vi "Return to Normal.vi"(8 "error in (no error)":errorcluster, 11 "Data Cluster in":T1 {"VestaTemperature"."Water Heater Temp (°F)" min=32 max=203}) -> (0 "error out":errorcluster, 1 "Send_Vesta_Message":u8, 3 "Data Cluster Output":T1 {"VestaTemperature"."Water Heater Temp (°F)" min=32 max=203})   [LabVIEW 2023]
uses:
  Drivers/Resideo Gas Valve/Type Definitions/Temperature Control.ctl
  Message Queue/Message Queue.lvlib
  Message Queue/Enqueue Message (Single).vi
  Drivers/Resideo Gas Valve/Type Definitions/Vesta Info.ctl
  controls/Burner Duty Cycle.ctl
  controls/Timer Application Cluster.ctl
  controls/UI Data.ctl
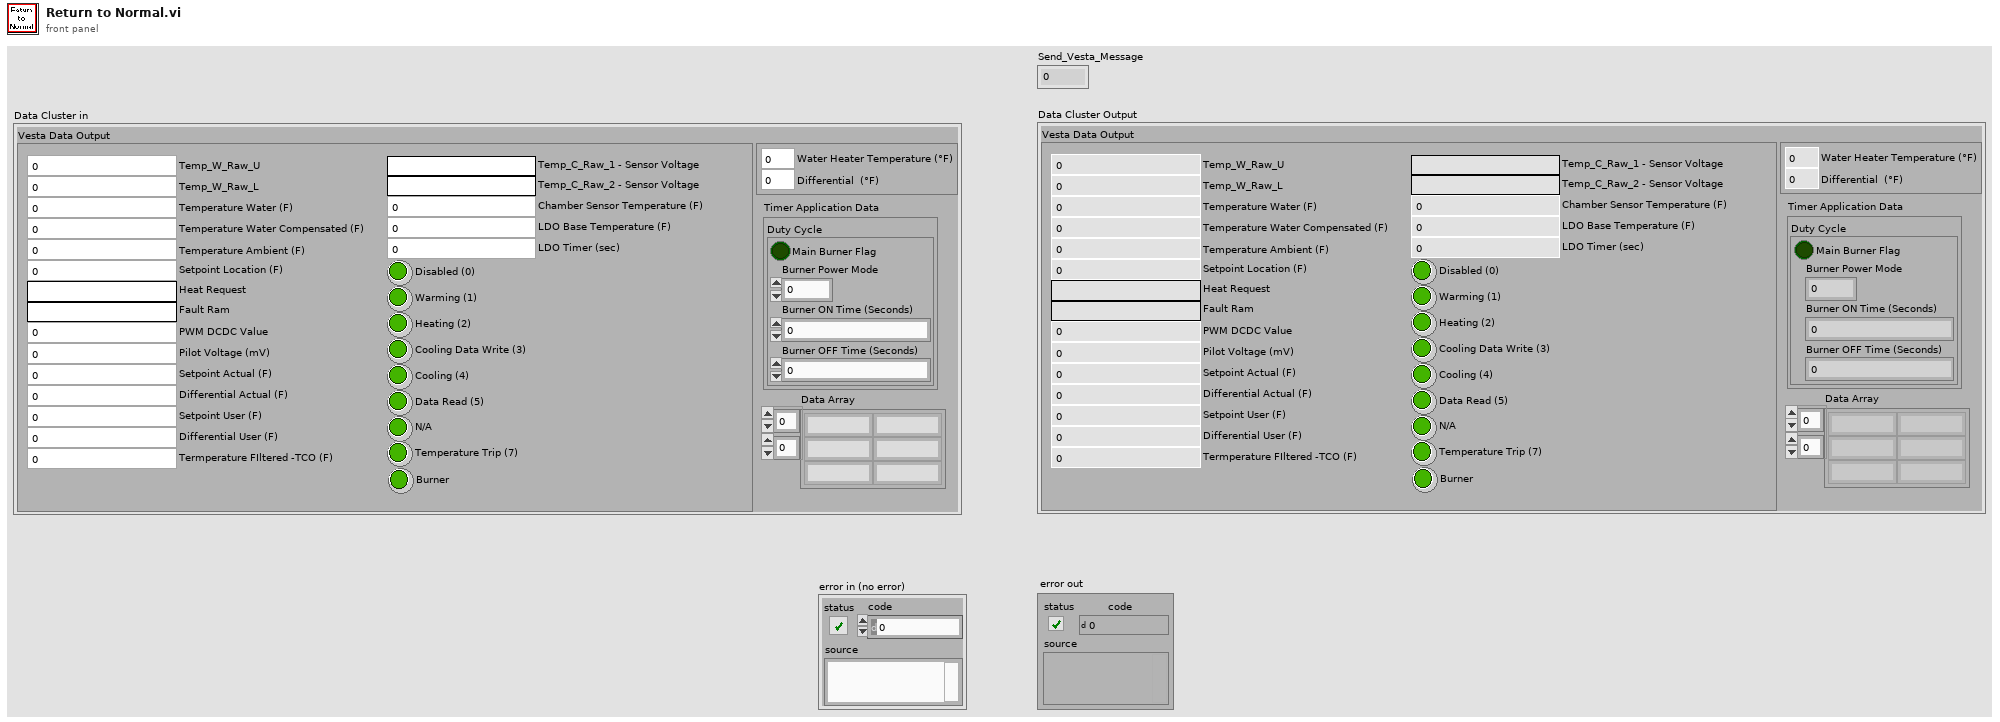
[diagram p1: front panel]
types:
  T1 = typedef "UI Data.ctl" = cluster{"Vesta Data Output":T2, "VestaTemperature":T3, "Timer Application Data":T4, "Data Array":string[][]}
  T2 = typedef "Vesta Info.ctl" = cluster{"Temp_W_Raw_U":u16, "Temp_W_Raw_L":u16, "Temperature Water (F)":dbl, "Temperature Water Compensated (F)":dbl, "Temperature Ambient (F)":dbl, "Setpoint Location (F)":dbl, "Heat Request":string, "Fault Ram":string, "PWM DCDC Value":u16, "Pilot Voltage (mV)":dbl, "Setpoint Actual (F)":dbl, "Differential Actual (F)":dbl, "Setpoint User (F)":dbl, "Differential User (F)":dbl, "Termperature FIltered -TCO (F)":dbl, "Temp_C_Raw_1 - Sensor Voltage":string, "Temp_C_Raw_2 - Sensor Voltage":string, "Chamber Sensor Temperature (F)":dbl, "LDO Base Temperature (F)":dbl, "LDO Timer (sec)":i16, "Disabled (0)":bool, "Warming (1)":bool, "Heating (2)":bool, "Cooling Data Write (3)":bool, "Cooling (4)":bool, "Data Read (5)":bool, "N/A":bool, "Temperature Trip (7)":bool, "Burner":bool}
  T3 = typedef "Temperature Control.ctl" = cluster{"Water Heater Temp (°F)":u16, "Differential  (°F)":dbl}
  T4 = typedef "Timer Application Cluster.ctl" = cluster{"Duty Cycle":T5}
  T5 = typedef "Burner Duty Cycle.ctl" = cluster{"Burner ON Time (Seconds)":dbl, "Burner OFF Time (Seconds)":dbl, "Main Burner Flag":bool, "Burner Power Mode":u8}
  T6 = typedef "UI Data.ctl" = cluster{"Vesta Data Output":T2, "VestaTemperature":T3, "Timer Application Data":T7}
  T7 = typedef "Timer Application Cluster.ctl" = cluster{"Time Data":T8, "Duty Cycle":T5}
  T8 = typedef "Timers.ctl" = cluster{"Main Timer":dbl, "Burner Status":bool}
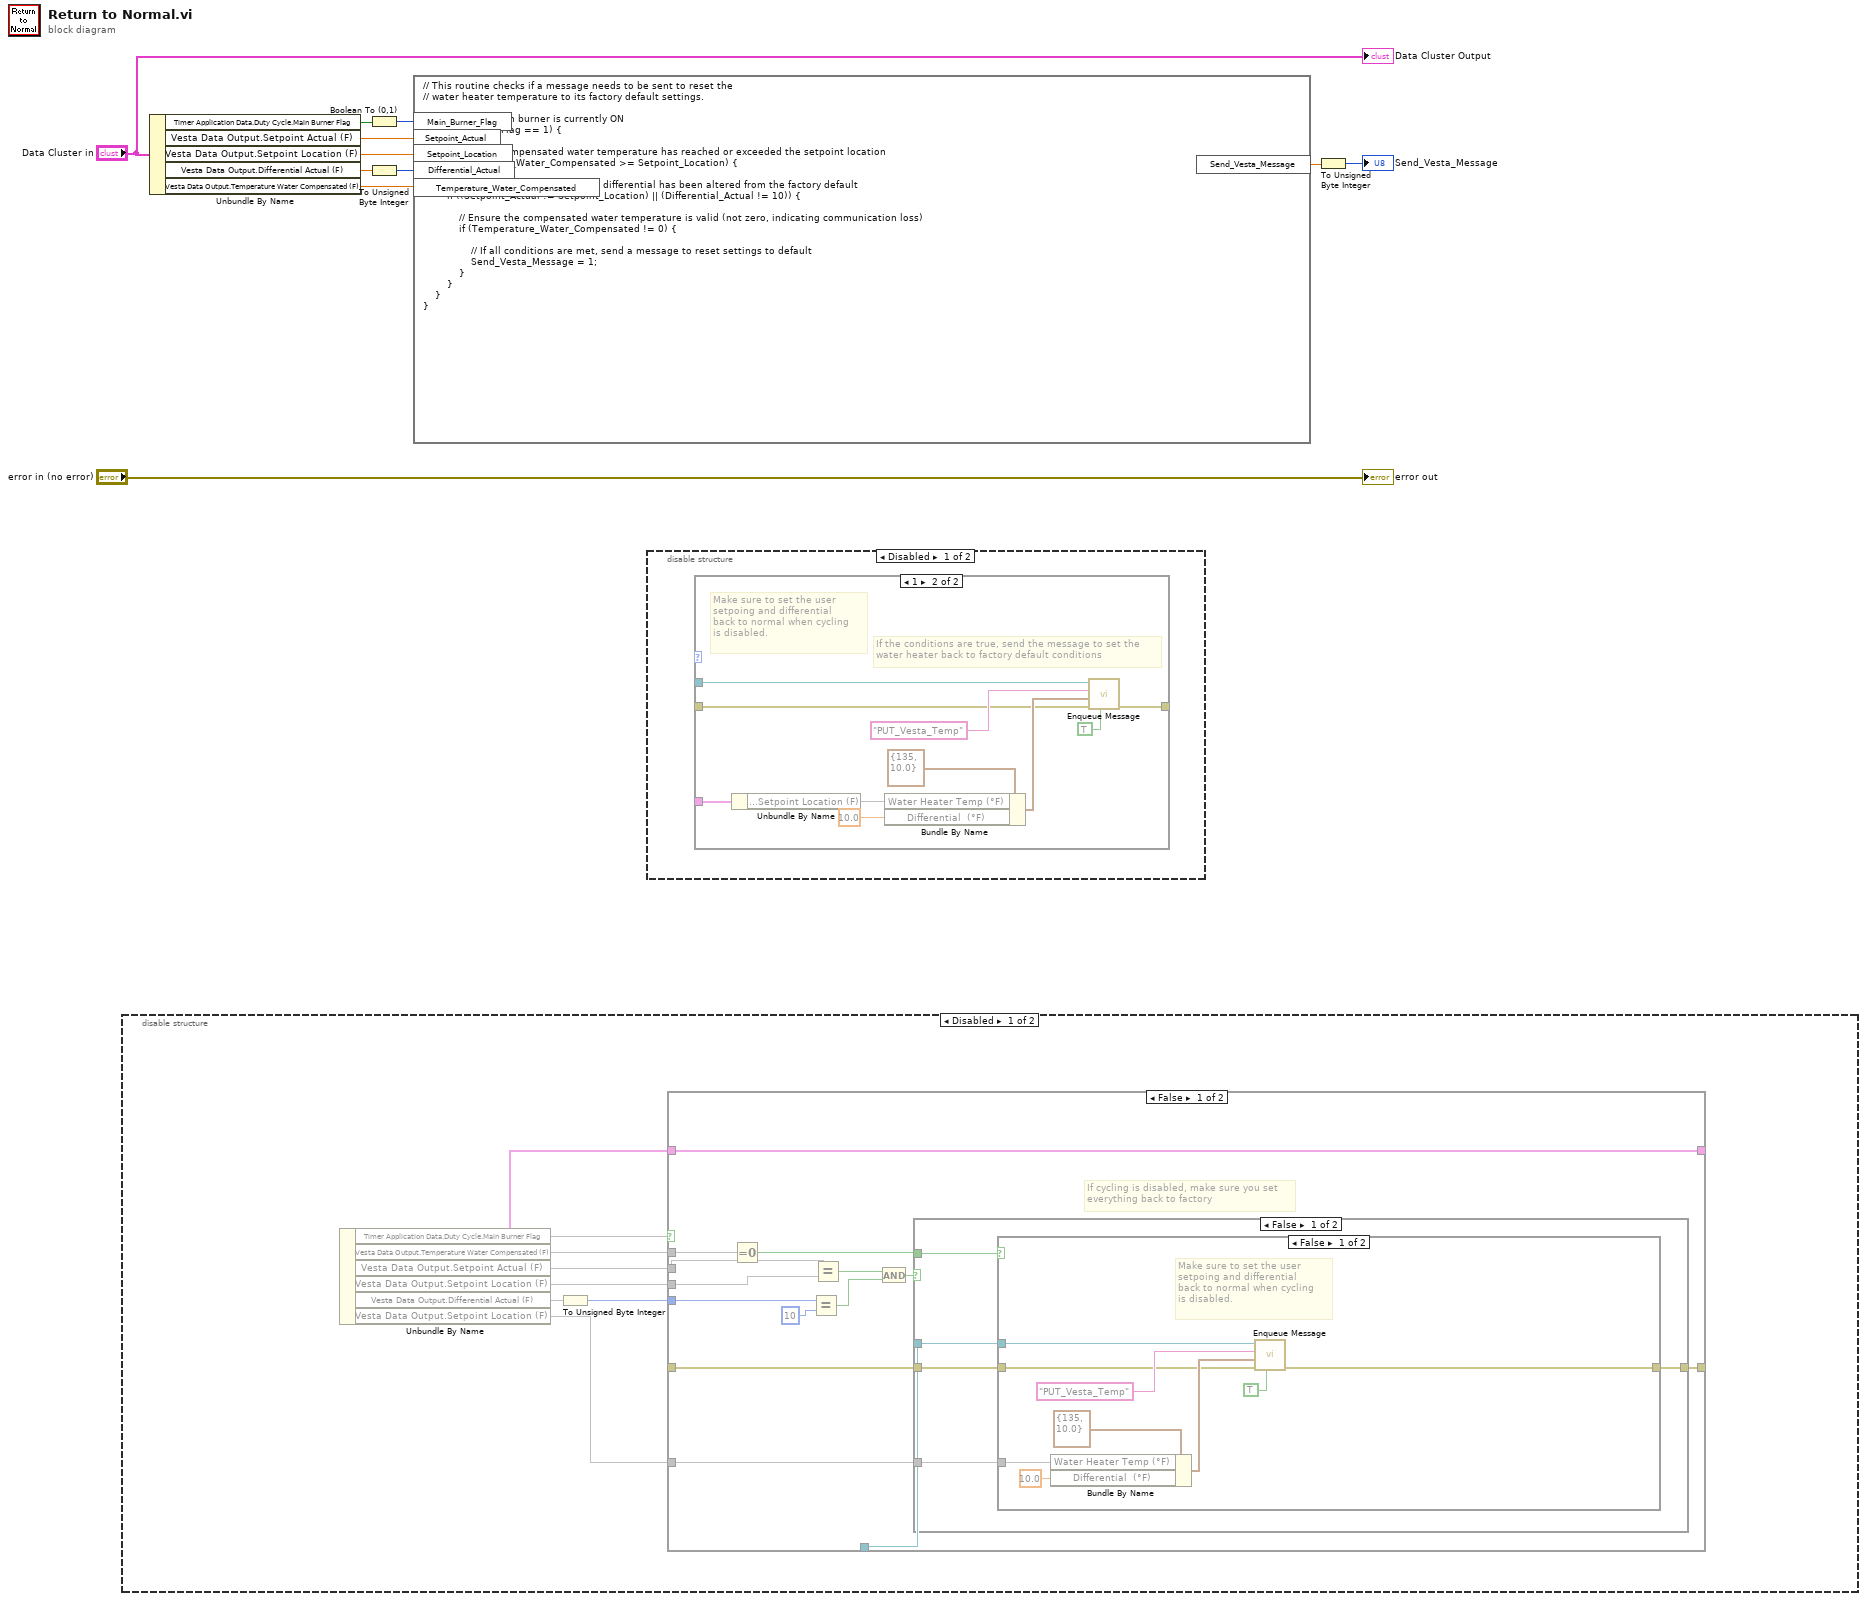
[diagram p0: block diagram]
diagram:
  n1 = disable-structure shown="Disabled" {
    frame Disabled {
      n2 = Unbundle By Name() -> (w19:T6, "Timer Application Data.Duty Cycle.Main Burner Flag"=w18, "Vesta Data Output.Temperature Water Compensated (F)"=w16, "Vesta Data Output.Setpoint Actual (F)"=w13, "Vesta Data Output.Setpoint Location (F)"=w12, "Vesta Data Output.Differential Actual (F)"=w14, "Vesta Data Output.Setpoint Location (F)"=w17)
      n3 = To Unsigned Byte Integer(number=w14) -> (unsigned 8bit integer=w15:u8)
      n4 = case shown="False" w18 {
        tunnel: _ -> [w33 _]
        tunnel: w15 -> [w31 _]
        tunnel: w13 -> [w30 _]
        tunnel: w12 -> [w29 _]
        tunnel: w17 -> [w28 _]
        tunnel: _ -> [w27 w51]
        tunnel: [w26 w51] -> _
        tunnel: w16 -> [w25 _]
        tunnel: w19 -> [w23 w50]
        tunnel: [w23 w50] -> _
        frame False {
          # "If cycling is disabled, make sure you set\neverything back to factory"
          n5 = Equal To 0?(x=w25) -> (x = 0?=w24:bool)
          n6 = Equal?(x=w31, y=u8 10) -> (x = y?=w21:bool)
          n7 = Equal?(x=w30, y=w29) -> (x = y?=w22:bool)
          n8 = And(x=w22, y=w21) -> (x .and. y?=w20:bool)
          n9 = case shown="False" w20 {
            tunnel: w33 -> [w38 _]
            tunnel: w28 -> [w37 _]
            tunnel: w27 -> [w36 w49]
            tunnel: [w35 w49] -> w26
            tunnel: w24 -> [w34 _]
            frame False {
              n10 = case shown="False" w34 {
                tunnel: w38 -> [w45 _]
                tunnel: w37 -> [w41 _]
                tunnel: w36 -> [w40 w48]
                tunnel: [w39 w48] -> w35
                frame False {
                  # "Make sure to set the user\nsetpoing and differential\nback to normal when cycling\nis disabled."
                  n11 = Bundle By Name(cluster=T3 {"Water Heater Temp (°F)"=135, "Differential  (°F)"=10.0} ("VestaTemperature"), "Water Heater Temp (°F)"=w41, "Differential  (°F)"=10.0) -> (w43:T3)
                  n12 = call-poly "Enqueue Message.vi"("Priority Message? (F)"=TRUE, "error in (no error)"=w40, "Message Data"=w43, "Message"="PUT_Vesta_Temp", "Message Queue"=w45) -> ("error out"=w39:errorcluster)  [unwired: 5 in, 1 out]
                }
                frame True {
                }
              }
            }
            frame True {
              # "Everything looks ok for the \nnone cycling mode"
            }
          }
        }
        frame True {
          # "If cycling is enabled, follow cycling routine."
        }
      }
    }
    frame Enabled {
    }
  }
  n13 = Unbundle By Name("Data Cluster in") -> ("Timer Application Data.Duty Cycle.Main Burner Flag"=w8:bool, "Vesta Data Output.Setpoint Actual (F)"=w7:dbl, "Vesta Data Output.Setpoint Location (F)"=w6:dbl, "Vesta Data Output.Differential Actual (F)"=w5:dbl, "Vesta Data Output.Temperature Water Compensated (F)"=w4:dbl)
  n14 = Boolean To (0,1)(Boolean=w8) -> (0, 1=w10:i16)
  n15 = To Unsigned Byte Integer(number=w5) -> (unsigned 8bit integer=w11:u8)
  n16 = formula code="// This routine checks if a message needs to be sent to reset the  \n// water heater temperature to its factory default settings.\n\n// Check if the main burner is currently ON\nif (Main_Burner_Flag == 1) {  \n\n    // Ensure the compensated water temperature has reached or exceeded the setpoint location\n    if (Temperature_Water_Compensated >= Setpoint_Location) {  \n\n        // Check if either the setpoint or differential has been altered from the factory default\n        if ((Setpoint_Actual != Setpoint_Location) || (Differential_Actual != 10)) {  \n\n            // Ensure the compensated water temperature is valid (not zero, indicating communication loss)\n            if (Temperature_Water_Compensated != 0) {  \n\n                // If all conditions are met, send a message to reset settings to default\n                Send_Vesta_Message = 1;  \n            }\n        }\n    }\n}"("Main_Burner_Flag"=w10, "Setpoint_Actual"=w7, "Setpoint_Location"=w6, "Differential_Actual"=w11, "Temperature_Water_Compensated"=w4) -> ("Send_Vesta_Message"=w9:dbl)
  n17 = disable-structure shown="Disabled" {
    frame Disabled {
      n18 = case shown="1" {
        selector: _ -> [_ _]
        tunnel: _ -> [_ w60]
        tunnel: _ -> [w52 w56]
        tunnel: [w52 w55] -> _
        tunnel: _ -> [_ w54]
        frame 0, Default {
        }
        frame 1 {
          # "If the conditions are true, send the message to set the \nwater heater back to factory default conditions"
          # "Make sure to set the user\nsetpoing and differential\nback to normal when cycling\nis disabled."
          n19 = Unbundle By Name(w54) -> ("Vesta Data Output.Setpoint Location (F)"=w53)
          n20 = Bundle By Name(cluster=T3 {"Water Heater Temp (°F)"=135, "Differential  (°F)"=10.0} ("VestaTemperature"), "Water Heater Temp (°F)"=w53, "Differential  (°F)"=10.0) -> (w58:T3)
          n21 = call-poly "Enqueue Message.vi"("Priority Message? (F)"=TRUE, "error in (no error)"=w56, "Message Data"=w58, "Message"="PUT_Vesta_Temp", "Message Queue"=w60) -> ("error out"=w55:errorcluster)  [unwired: 5 in, 1 out]
        }
      }
    }
    frame Enabled {
    }
  }
  n22 = To Unsigned Byte Integer(number=w9) -> (unsigned 8bit integer=→"Send_Vesta_Message":u8)
  "error out" <- "error in (no error)"
  "Data Cluster Output" <- "Data Cluster in"
